vi "Write REF Filter.vi"(8 "error in (no error)":errorcluster, 10 "Configuration.REF Filter.REF filter":T1={"TC (s)"=0.3, "order"=2} {"TC (s)" format="%#_6p"}, 11 "Instrument.Lockin in":refnum<class "Instrument.Lockin.lvclass">) -> (0 "error out":errorcluster, 3 "Instrument.Lockin out":refnum<class "Instrument.Lockin.lvclass">)   [LabVIEW 2016, in "Instrument.Lockin.lvclass"]
uses:
  Instrument.Lockin.lvclass
  LockinDAQ/Typedefs/REF filter-cluster.ctl
  Instrument.Lockin.lvclass/Instrument.Lockin.ctl
  LockinDAQ/LockinDAQ.lvclass
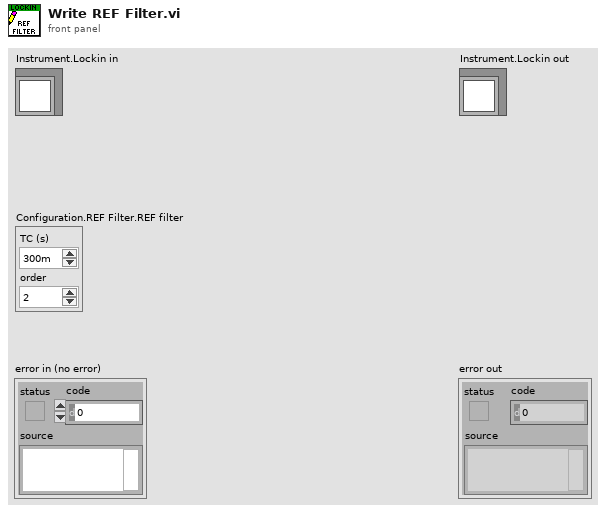
[diagram p1: front panel]
types:
  T1 = typedef "LockinDAQ.lvclass/REF filter-cluster.ctl" = cluster{"TC (s)":dbl, "order":i32}
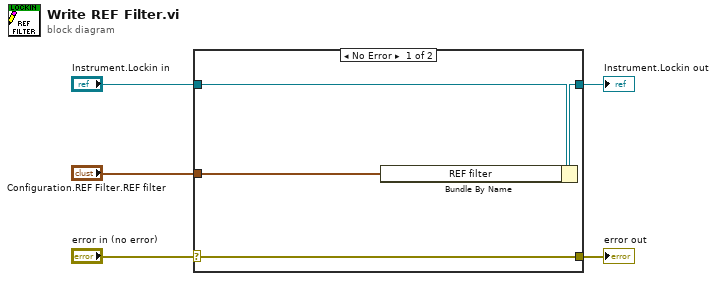
[diagram p0: block diagram]
diagram:
  n1 = case shown="No Error" "error in (no error)" {
    selector: "error in (no error)" -> [w9 w10]
    tunnel: [w9 w10] -> w4
    tunnel: [w7 w11] -> w2
    tunnel: "Instrument.Lockin in" -> [w8 w11]
    tunnel: "Configuration.REF Filter.REF filter" -> [w6 _]
    frame No Error {
      n2 = Bundle By Name(cluster=w8, "REF filter"=w6) -> (w7:refnum<class "Instrument.Lockin.lvclass">)
    }
    frame Error {
    }
  }
  "error out" <- w4
  "Instrument.Lockin out" <- w2
